vi "Hours.vi"(8 "error in (no error)":errorcluster, 10 "base path":path, 11 "Names":string[](array[string])) -> (0 "error out":errorcluster)   [LabVIEW 2020]
uses:
  controls/Names.ctl
  System.Windows.Forms
  controls/Report Cases.ctl
  <vilib>/Utility/error.llb/DialogType.ctl
panel:
  out "Total Time":string
  in  "Email Address":string caption="Recipients"
  in  "Mail Button":bool
  in  "Find Data":bool
  in  "OK Button":bool
  in  "To":refnum<k24>(container)
  in  "From":refnum<k24>(container)
  in  "Name":T1 items=["Adriana Chou", "Austin Scholp", "Boquan Liu", "Colin Schrof", "David Piotrowski", "Evan Polce", "Hayley Raj", "Hunter Bourne", "Hunter Huth", "Jack Ersbo", "Jack J", "Jacob Tangney", "Jake Reiss", "Jennifer German", "Jessica Wang", "JJ Lamb", "Lifan Yu", "Wyatt Barber"]
  out "Report Data":string[][](array[string])
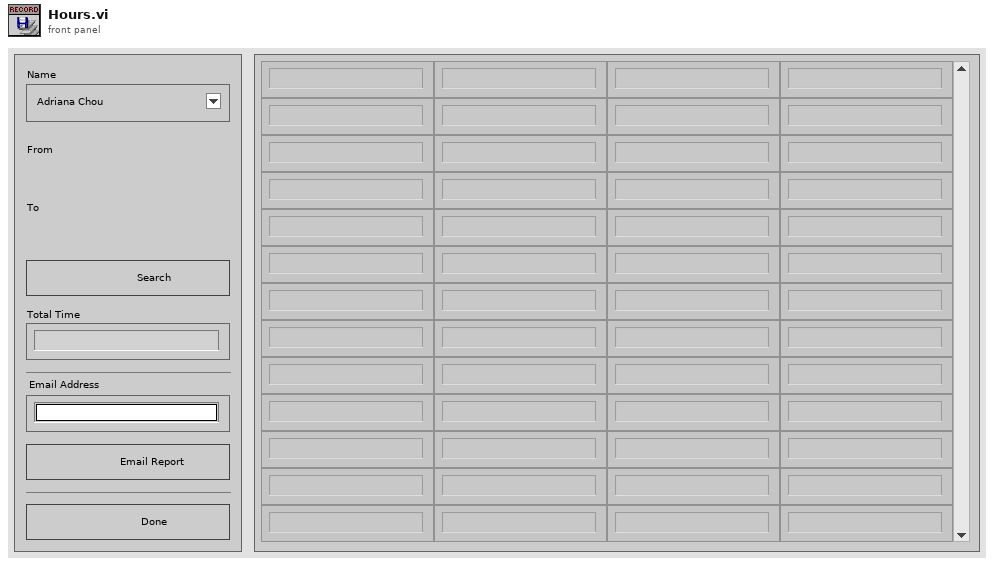
[diagram p1: front panel]
types:
  T1 = typedef "Names.ctl" = u16
  T2 = enum16{"open", "replace", "create", "open or create", "replace or create", "replace or create with confirmation"}
  T3 = typedef "Report Cases.ctl" = enum16{"Wait", "Search", "Email", "Full Report", "Exit"}
  T4 = typedef "eventvkey.ctl" = enum16{"ASCII", "Enter", "Return", "Shift", "Ctrl", "Alt", "Cmd", "Opt", "Caps", "NumLock", "Clear", "Break", "Up", "Down", "Left", "Right", "Insert", "Delete", "Home", "End", "PageUp", "PageDown", "Escape", "Help", "Pause", "ScrollLock", "F1", "F2", "F3", "F4", "F5", "F6", "F7", "F8", "F9", "F10", "F11", "F12", "F13", "F14", "F15", "F16", "F17", "F18", "F19", "F20", "F21", "F22", "F23", "F24", "Play", "VolumeUp", "VolumeDown", "Mute", "Two Byte Char"}
  T5 = typedef "DialogType.ctl" = u16
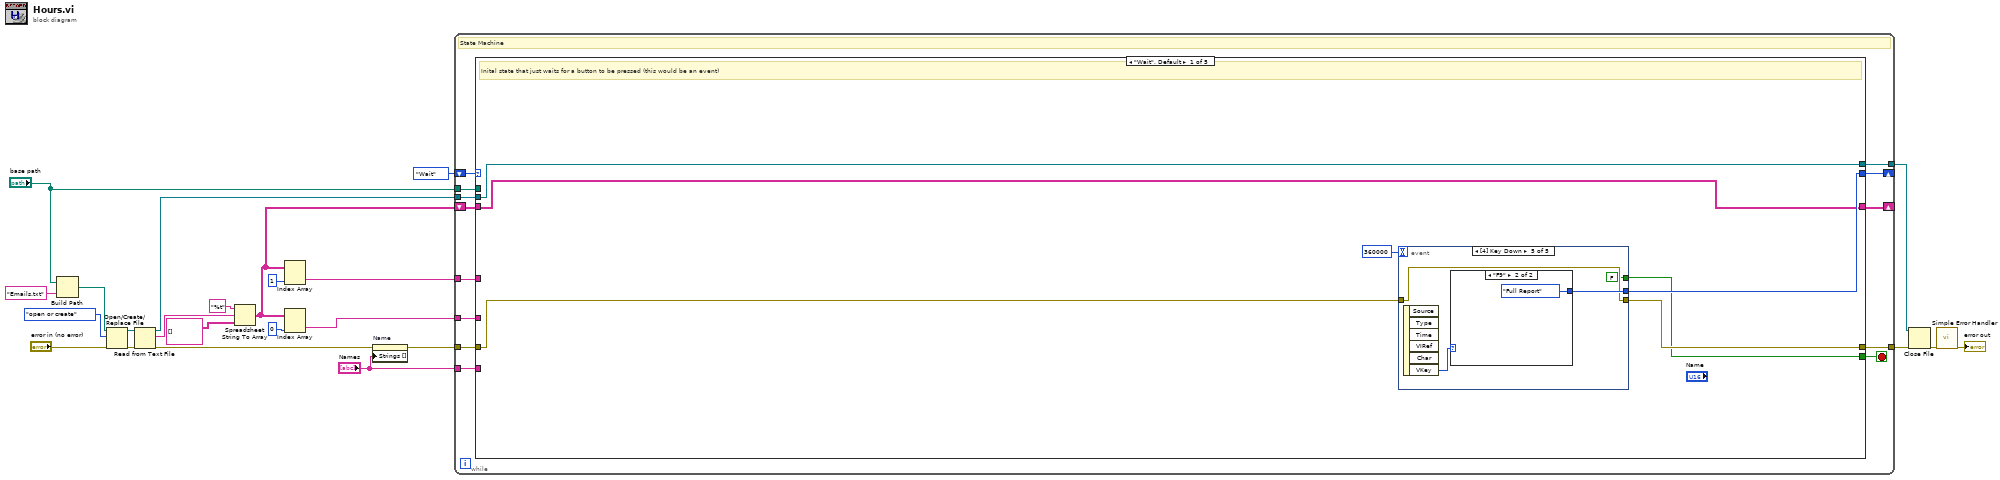
[diagram p0: block diagram]
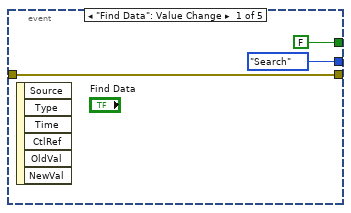
[diagram p2: hidden frame]
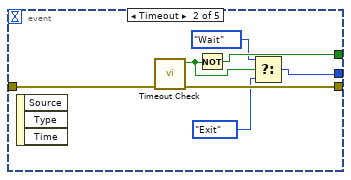
[diagram p3: hidden frame]
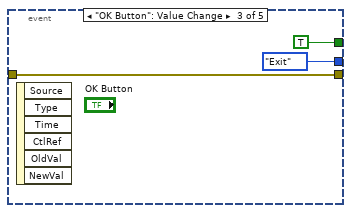
[diagram p4: hidden frame]
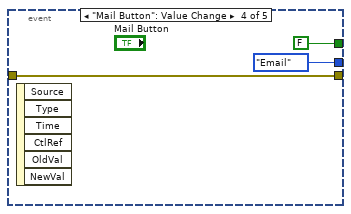
[diagram p5: hidden frame]
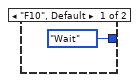
[diagram p6: hidden frame]
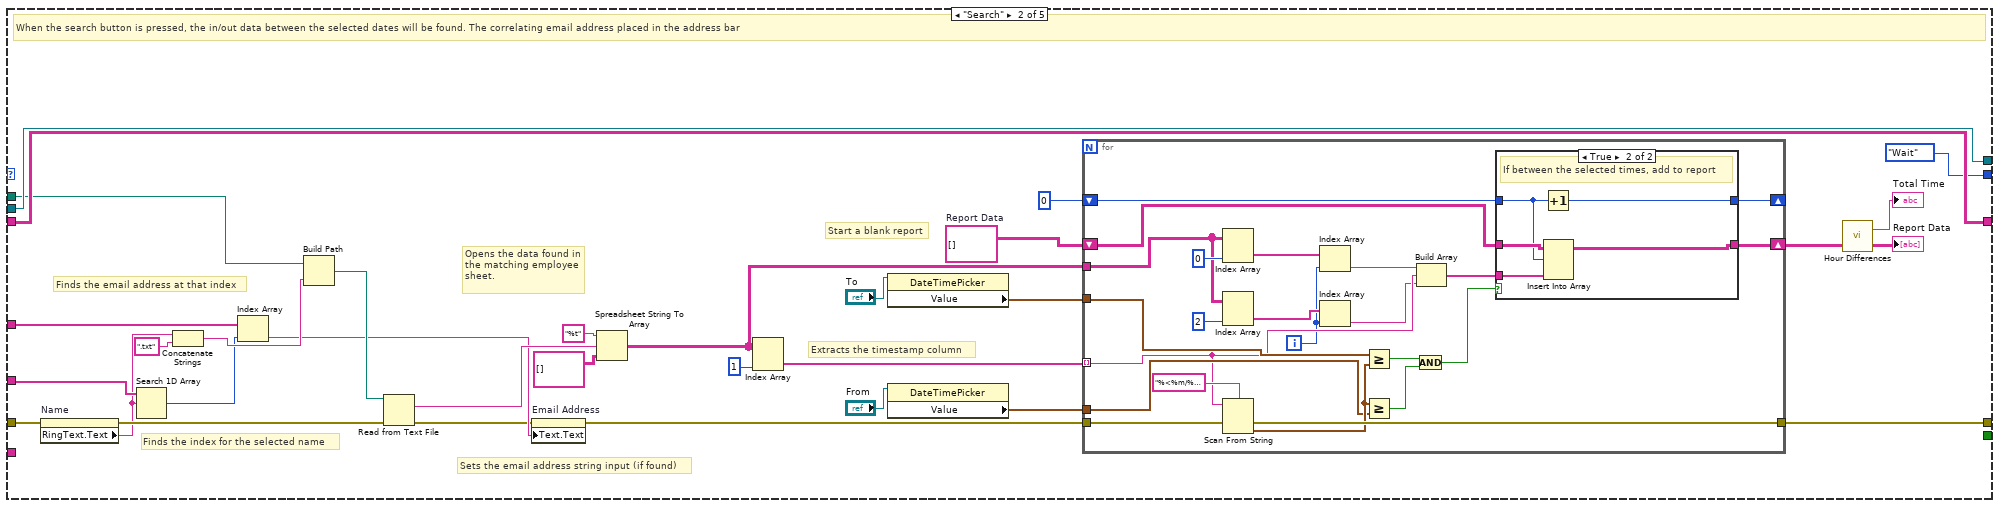
[diagram p7: hidden frame]
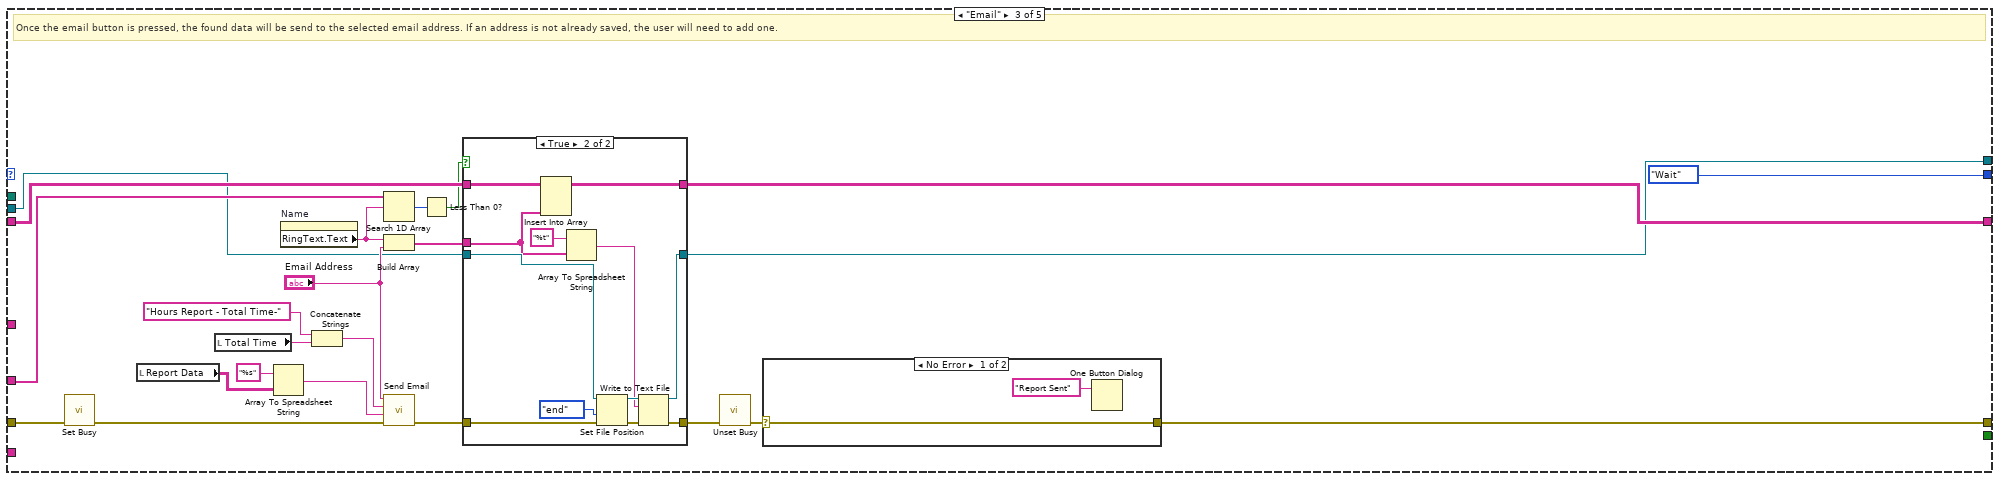
[diagram p9: hidden frame]
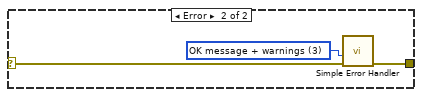
[diagram p11: hidden frame]
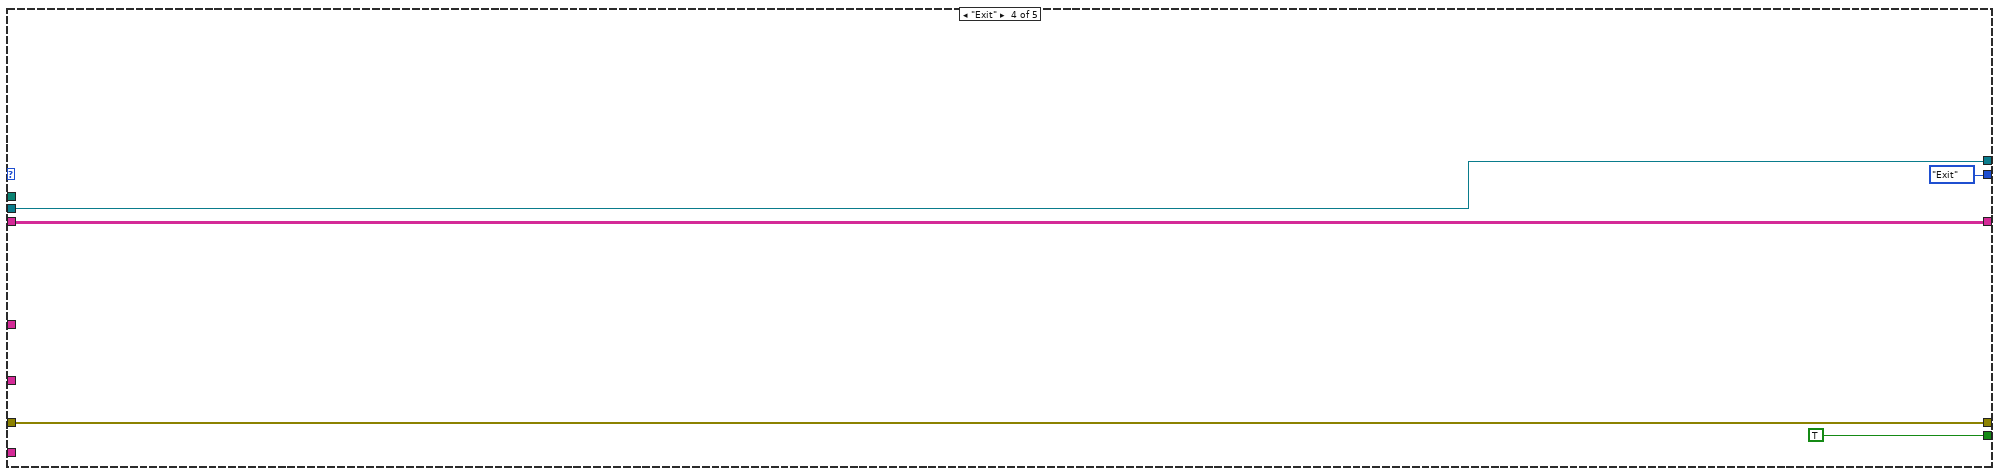
[diagram p12: hidden frame]
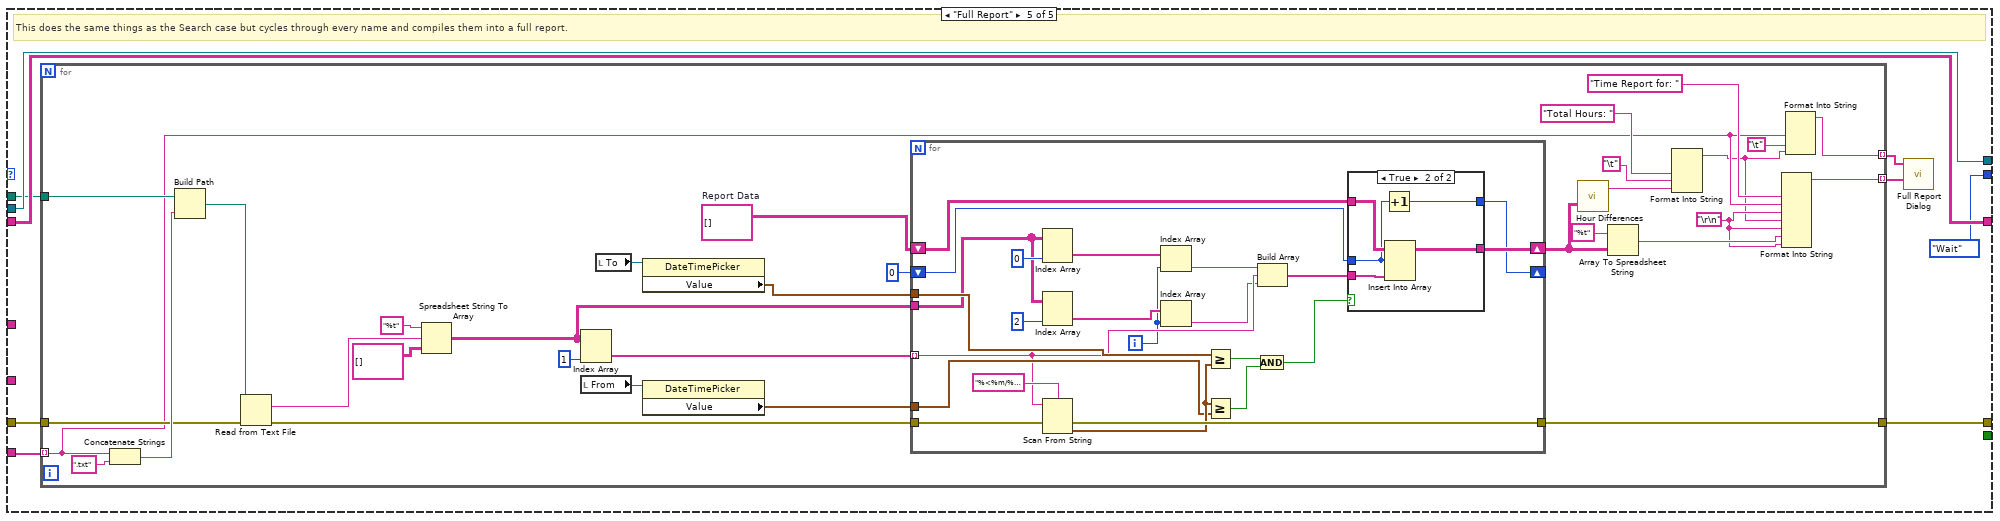
[diagram p13: hidden frame]
diagram:
  n1 = Build Path(base path="base path", name or relative path="Emails.txt") -> (appended path=w2:path)
  n2 = Open/Create/Replace File(file path (use dialog)=w2, error in="error in (no error)", operation (0:open)=T2."open or create") -> (refnum out=w16:refnum<file>, error out=w19:errorcluster)  [unwired: 3 in, 1 out]
  n3 = Read from Text File(file (use dialog)=w16, error in=w19) -> (refnum out=w11:refnum<file>, text=w18:string, error out=w17:errorcluster)  [unwired: 2 in, 1 out]
  n4 = Spreadsheet String To Array(format string="%t", spreadsheet string=w18, array type (2D Dbl)=string[][] []) -> (array=w8:string[][])  [unwired: 1 in]
  n5 = Index Array(array=w8, index (col)=1 ("disabled index (col)")) -> (element=w12:string[])  [unwired: 1 in]
  n6 = Index Array(array=w8, index (col)=0 ("disabled index (col)")) -> (element=w14:string[])  [unwired: 1 in]
  n7 = property on="Name" class="Ring (strict)"(error in=w17, "Strings []"="Names") -> (error out=w23:errorcluster)  [unwired: 1 in, 1 out]
  n8 = while {
    shift-right: [w36] -> _
    shift-left: Report_Cases."Wait" -> [w33]
    tunnel: w23 -> [w37]
    tunnel: [w35] -> w10
    tunnel: w14 -> [w32]
    tunnel: w12 -> [w31]
    tunnel: w11 -> [w30]
    tunnel: [w29] -> w9
    shift-right: [w27] -> _
    shift-left: w8 -> [w28]
    tunnel: "Names" -> [w26]
    tunnel: "base path" -> [w25]
    stop <- w34 stop-if-true
    # "State Machine"
    n9 = case shown="\"Wait\", Default" w33 {
      tunnel: w37 -> [w44 w91 w144 w175 w185]
      tunnel: [w42 Report_Cases."Wait" Report_Cases."Wait" Report_Cases."Exit" Report_Cases."Wait"] -> w36
      tunnel: [w43 w88 w141 w175 w184] -> w35
      tunnel: [w41 _ _ TRUE _] -> w34
      tunnel: w32 -> [_ w84 w140 _ _]
      tunnel: w31 -> [_ w82 _ _ _]
      tunnel: w30 -> [w40 w77 w135 w174 w182]
      tunnel: [w40 w77 w134 w174 w182] -> w29
      tunnel: w28 -> [w39 w72 w145 w173 w183]
      tunnel: [w39 w72 w139 w173 w183] -> w27
      tunnel: w26 -> [_ _ _ _ w179]
      tunnel: w25 -> [_ w68 _ _ w178]
      frame "Wait", Default {
        # "Inital state that just waits for a button to be pressed (this would be an event)"
        n10 = event shown="[4] Key Down" {
          selector: _ -> [_ _ _ _ _]
          dyn-events: _ -> [_ _ _ _ _]
          timeout: 360000 -> [_ _ _ _ _]
          tunnel: w44 -> [w47 w54 w56 w59 w62]
          tunnel: [w47 w53 w56 w59 w62] -> w43
          tunnel: [Report_Cases."Search" w48 Report_Cases."Exit" Report_Cases."Email" w63] -> w42
          tunnel: [FALSE w52 TRUE FALSE FALSE] -> w41
          event "Find Data": Value Change {
            n11 = event-data() -> ()  [unwired: 1 in, 6 out]
          }
          event Timeout {
            n12 = event-data() -> ()  [unwired: 1 in, 3 out]
            n13 = call "Timeout Check.vi"("Error In"=w54) -> ("Error Out"=w53:errorcluster, "Still there?"=w51:bool)  [unwired: 9 in]
            n14 = Not(x=w51) -> (.not. x?=w52:bool)
            n15 = Select(t=Report_Cases."Wait", s=w51, f=Report_Cases."Exit") -> (s? t:f=w48:T3)
          }
          event "OK Button": Value Change {
            n16 = event-data() -> ()  [unwired: 1 in, 6 out]
          }
          event "Mail Button": Value Change {
            n17 = event-data() -> ()  [unwired: 1 in, 6 out]
          }
          event Key Down {
            n18 = event-data() -> ("VKey"=w64:T4)  [unwired: 1 in, 5 out]
            n19 = case shown="\"F9\"" w64 {
              tunnel: [Report_Cases."Wait" Report_Cases."Full Report"] -> w63
              frame "F10", Default {
              }
              frame "F9" {
              }
            }
          }
        }
      }
      frame "Search" {
        w85 = string[][] []  # Report Data
        # "Start a blank report"
        # "Extracts the timestamp column"
        # "Opens the data found in the matching employee sheet."
        # "Finds the email address at that index"
        # "Sets the email address string input (if found)"
        # "Finds the index for the selected name"
        # "When the search button is pressed, the in/out data between the selected dates will be found. The correlating email address placed in the address bar"
        n20 = property on="Name" class="Ring (strict)"(error in=w91) -> (error out=w94:errorcluster, "RingText.Text"=w83:string)  [unwired: 1 in, 1 out]
        n21 = Search 1D Array(1D array=w84, element=w83) -> (index of element=w81:i32)  [unwired: 1 in]
        n22 = Concatenate Strings(w83, ".txt" ("string")) -> (w92:string)
        n23 = Index Array "Index Array"(array=w82, index=w81) -> (element=w80:string)
        n24 = Build Path(base path=w68, name or relative path=w92) -> (appended path=w95:path)
        n25 = Read from Text File(file (use dialog)=w95, error in=w94) -> (text=w96:string, error out=w79:errorcluster)  [unwired: 2 in, 2 out]
        n26 = property on="Email Address" class="Str"(error in=w79, "Text.Text"=w80) -> (error out=w78:errorcluster)  [unwired: 1 in, 1 out]
        n27 = Spreadsheet String To Array(format string="%t", spreadsheet string=w96, array type (2D Dbl)=string[][] []) -> (array=w74:string[][])  [unwired: 1 in]
        n28 = Index Array "Index Array"(array=w74, index (col)=1 ("disabled index (col)")) -> (element=w75:string[])  [unwired: 1 in]
        n29 = property class="DateTimePicker"(reference="To") -> ("Value"=w87:timestamp)  [unwired: 1 in, 2 out]
        n30 = property class="DateTimePicker"(reference="From") -> ("Value"=w86:timestamp)  [unwired: 1 in, 2 out]
        n31 = for {
          tunnel: w78 -> [w121]
          tunnel: [w120] -> w88
          shift-right: [w118] -> w71
          shift-left: w85 -> [w119]
          tunnel: w86 -> [w111]
          tunnel: w87 -> [w116]
          tunnel: w75 -> [w109] mode=indexing
          tunnel: w74 -> [w102]
          shift-right: [w104] -> _
          shift-left: 0 -> [w105]
          i -> [w99]
          n32 = Index Array "Index Array"(array=w102, index (col)=0) -> (element=w107:string[])  [unwired: 1 in]
          n33 = Index Array "Index Array"(array=w102, index (col)=2 ("disabled index (col)")) -> (element=w103:string[])  [unwired: 1 in]
          n34 = Scan From String "Scan From String"(format string="%<%m/%d/%Y %I:%M:%S%3u %p>T", input string=w109, error in=w121) -> (error out=w120:errorcluster, output 1=w113:timestamp)  [unwired: 2 in, 2 out]
          n35 = Index Array "Index Array"(array=w107, index=w99) -> (element=w106:string)
          n36 = Index Array "Index Array"(array=w103, index=w99) -> (element=w100:string)
          n37 = Greater Or Equal?(x=w116, y=w113) -> (x >= y?=w115:bool)
          n38 = Greater Or Equal?(x=w113, y=w111) -> (x >= y?=w112:bool)
          n39 = And(x=w115, y=w112) -> (x .and. y?=w114:bool)
          n40 = Build Array "Build Array"(w106, w109, w100) -> (w110:string[])
          n41 = case shown="True" w114 {
            tunnel: w119 -> [w123 w128]
            tunnel: [w123 w127] -> w118
            tunnel: w110 -> [_ w126]
            tunnel: w105 -> [w122 w124]
            tunnel: [w122 w125] -> w104
            frame False {
              # "If outside selected times, do nothing"
            }
            frame True {
              # "If between the selected times, add to report"
              n42 = Increment(x=w124) -> (x+1=w125:i32)
              n43 = Insert Into Array "Insert Into Array"(array=w128, index (row)=w124, new element=w126) -> (w127:string[][])  [unwired: 1 in]
            }
          }
        }
        n44 = call "Hour Differences.vi"("Report Data In"=w71) -> ("Report Data Out"=→"Report Data":string[][], "Total Hours"=→"Total Time":string)  [unwired: 1 in]
      }
      frame "Email" {
        # "Once the email button is pressed, the found data will be send to the selected email address. If an address is not already saved, the user will need to add one."
        n45 = call <vilib>:"Set Busy.vi"("error in (no error)"=w144) -> ("error out"=w143:errorcluster)  [unwired: 9 in, 1 out]
        n46 = local read "Report Data"() -> (w150:string[][])
        n47 = local read "Total Time"() -> (w130:string)
        n48 = Array To Spreadsheet String(array=w150, 3:"%s" ("format string")) -> (spreadsheet string=w148:string)  [unwired: 1 in]
        n49 = property on="Name" class="Ring (strict)"() -> ("RingText.Text"=w147:string)  [unwired: 2 in, 2 out]
        n50 = Concatenate Strings("Hours Report - Total Time-" ("Subject"), w130) -> (w129:string)
        n51 = Search 1D Array(1D array=w140, element=w147) -> (index of element=w138:i32)  [unwired: 1 in]
        n52 = Build Array(w147, "Email Address") -> (w146:string[])
        n53 = call "Send Email"("error in"=w143, "Message"=w148, "Subject"=w129, "Recipients"="Email Address") -> ("error out"=w132:errorcluster)  [unwired: 7 in]
        n54 = Less Than 0?(x=w138) -> (x < 0?=w137:bool)
        n55 = case shown="True" w137 {
          tunnel: w146 -> [_ w157]
          tunnel: w145 -> [w154 w166]
          tunnel: [w154 w165] -> w139
          tunnel: w135 -> [w153 w163]
          tunnel: [w153 w161] -> w134
          tunnel: [w152 w160] -> w133
          tunnel: w132 -> [w152 w159]
          frame False {
          }
          frame True {
            n56 = Insert Into Array(array=w166, new element=w157) -> (w165:string[][])  [unwired: 2 in]
            n57 = Array To Spreadsheet String(array=w157, 3:"%t" ("format string")) -> (spreadsheet string=w156:string)  [unwired: 1 in]
            n58 = Set File Position(refnum=w163, from (0:start)=enum16{"start", "end", "current"}."end", error in=w159) -> (refnum out=w162:refnum<file>, error out=w158:errorcluster)  [unwired: 1 in]
            n59 = Write to Text File(file (use dialog)=w162, text=w156, error in=w158) -> (refnum out=w161:refnum<file>, error out=w160:errorcluster)  [unwired: 1 in, 1 out]
          }
        }
        n60 = call <vilib>:"Unset Busy.vi"("error in (no error)"=w133) -> ("error out"=w142:errorcluster)  [unwired: 10 in]
        n61 = case shown="No Error" w142 {
          selector: w142 -> [w167 w171]
          tunnel: [w167 w170] -> w141
          frame No Error {
            n62 = One Button Dialog(message="Report Sent") -> ()  [unwired: 1 in, 1 out]
          }
          frame Error {
            w169 = T5 3 items=["no dialog", "OK message", "continue or stop message", "OK message + warnings", "continue/stop + warnings"] ("type of dialog (OK msg:1)")
            n63 = call <vilib>:"Simple Error Handler.vi"("type of dialog (OK msg:1)"=w169, "error in (no error)"=w171) -> ("error out"=w170:errorcluster)  [unwired: 3 in, 4 out]
          }
        }
      }
      frame "Exit" {
      }
      frame "Full Report" {
        # "This does the same things as the Search case but cycles through every name and compiles them into a full report."
        n64 = for {
          tunnel: w185 -> [w201]
          tunnel: w179 -> [w190] mode=indexing
          tunnel: [w200] -> w184
          tunnel: [w186] -> w181 mode=indexing
          tunnel: [w199] -> w180 mode=indexing
          tunnel: w178 -> [w196]
          w188 = "\r\n"
          w209 = string[][] []  # Report Data
          n65 = Concatenate Strings(w190, ".txt" ("string")) -> (w212:string)
          n66 = Build Path(base path=w196, name or relative path=w212) -> (appended path=w214:path)
          n67 = Read from Text File(file (use dialog)=w214, error in=w201) -> (text=w215:string, error out=w202:errorcluster)  [unwired: 2 in, 2 out]
          n68 = Spreadsheet String To Array(format string="%t", spreadsheet string=w215, array type (2D Dbl)=string[][] []) -> (array=w208:string[][])  [unwired: 1 in]
          n69 = Index Array "Index Array"(array=w208, index (col)=1 ("disabled index (col)")) -> (element=w206:string[])  [unwired: 1 in]
          n70 = local read "From"() -> (w203:refnum<k24>)
          n71 = local read "To"() -> (w204:refnum<k24>)
          n72 = property class="DateTimePicker"(reference=w204) -> ("Value"=w207:timestamp)  [unwired: 1 in, 2 out]
          n73 = property class="DateTimePicker"(reference=w203) -> ("Value"=w205:timestamp)  [unwired: 1 in, 2 out]
          n74 = for {
            tunnel: w202 -> [w240]
            tunnel: [w239] -> w200
            shift-right: [w237] -> w197
            shift-left: w209 -> [w238]
            tunnel: w205 -> [w230]
            tunnel: w207 -> [w235]
            tunnel: w206 -> [w228] mode=indexing
            tunnel: w208 -> [w221]
            shift-right: [w223] -> _
            shift-left: 0 -> [w224]
            i -> [w218]
            n75 = Index Array "Index Array"(array=w221, index (col)=0) -> (element=w226:string[])  [unwired: 1 in]
            n76 = Index Array "Index Array"(array=w221, index (col)=2 ("disabled index (col)")) -> (element=w222:string[])  [unwired: 1 in]
            n77 = Scan From String "Scan From String"(format string="%<%m/%d/%Y %I:%M:%S%3u %p>T", input string=w228, error in=w240) -> (error out=w239:errorcluster, output 1=w232:timestamp)  [unwired: 2 in, 2 out]
            n78 = Index Array "Index Array"(array=w226, index=w218) -> (element=w225:string)
            n79 = Index Array "Index Array"(array=w222, index=w218) -> (element=w219:string)
            n80 = Greater Or Equal?(x=w235, y=w232) -> (x >= y?=w234:bool)
            n81 = Greater Or Equal?(x=w232, y=w230) -> (x >= y?=w231:bool)
            n82 = And(x=w234, y=w231) -> (x .and. y?=w233:bool)
            n83 = Build Array "Build Array"(w225, w228, w219) -> (w229:string[])
            n84 = case shown="True" w233 {
              tunnel: w238 -> [w242 w247]
              tunnel: [w242 w246] -> w237
              tunnel: w229 -> [_ w245]
              tunnel: w224 -> [w241 w243]
              tunnel: [w241 w244] -> w223
              frame False {
              }
              frame True {
                n85 = Increment(x=w243) -> (x+1=w244:i32)
                n86 = Insert Into Array "Insert Into Array"(array=w247, index (row)=w243, new element=w245) -> (w246:string[][])  [unwired: 1 in]
              }
            }
          }
          n87 = call "Hour Differences.vi"("Report Data In"=w197) -> ("Total Hours"=w193:string)  [unwired: 1 in, 1 out]
          n88 = Array To Spreadsheet String(array=w197, 3:"%t" ("format string")) -> (spreadsheet string=w191:string)  [unwired: 1 in]
          n89 = Format Into String("Total Hours: " ("string"), "\t", w193) -> (resulting string=w187:string)  [unwired: 3 in, 1 out]
          n90 = Format Into String("Time Report for: " ("string"), w190, w188, w187, w188, w191, w188) -> (resulting string=w199:string)  [unwired: 3 in, 1 out]
          n91 = Format Into String(w190, "\t", w187) -> (resulting string=w186:string)  [unwired: 3 in, 1 out]
        }
        n92 = call "Full Report Dialog.vi"("Time Reports In"=w180, "Total Hours In"=w181) -> ()  [unwired: 10 in]
      }
    }
  }
  n93 = Close File(refnum=w9, error in=w10) -> (error out=w6:errorcluster)  [unwired: 1 out]
  n94 = call <vilib>:"Simple Error Handler.vi"("error in (no error)"=w6) -> ("error out"=→"error out":errorcluster)  [unwired: 4 in, 4 out]
